vi "Set Zero Offset Mode.vi"(8 "error in (no error)":errorcluster, 9 "Reference Value (0.0)":dbl format="%.4f", 10 "Zero Offset Mode (F: Off)":bool, 11 "VISA resource name":refnum<visa-resource-name>) -> (0 "error out":errorcluster, 3 "VISA resource name out":refnum<visa-resource-name>)   [LabVIEW 2014, in "Fluke 5XXX Series Multicalibrators.lvlib"]
doc: "This VI zeros the pressure module or sets the zero offset for capacitance measurement using the oscilloscope option. For pressure measurments, if the pressure module is an absolute module, the reference parameter must be supplied.\n\nNote:\n\nThis VI is available only for instrument models 5500A and 5520A with oscilloscope option SC600 (SC1100) or option 700P (pressure modules)."
uses:
  Fluke 5XXX Series Multicalibrators.lvlib
panel:
  # "On"
  # "Off"
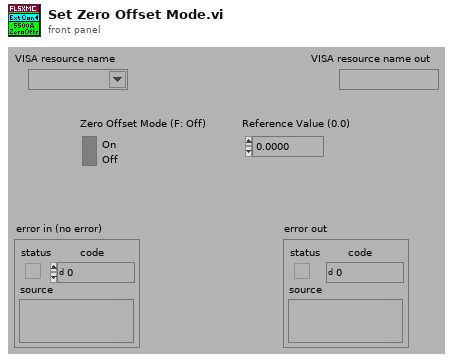
[diagram p1: front panel]
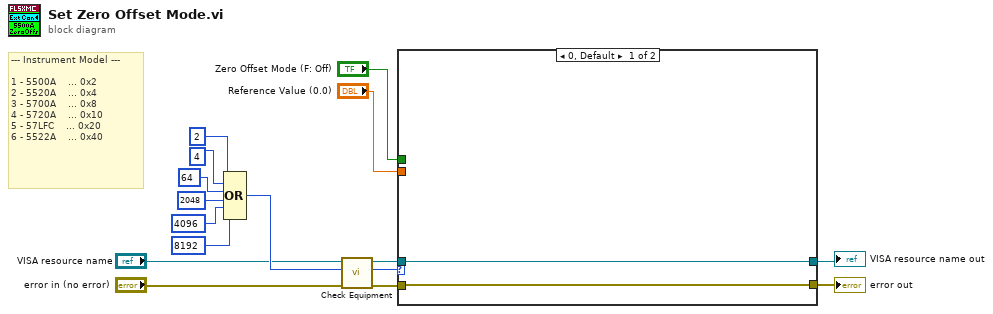
[diagram p0: block diagram]
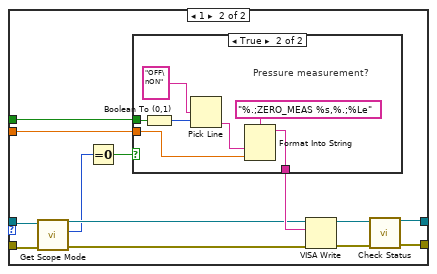
[diagram p2: hidden frame]
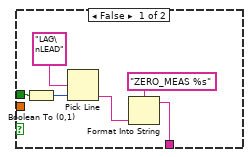
[diagram p3: hidden frame]
diagram:
  # "--- Instrument Model ---\n\n1 - 5500A    ... 0x2\n2 - 5520A    ... 0x4\n3 - 5700A    ... 0x8\n4 - 5720A    ... 0x10\n5 - 57LFC    ... 0x20\n6 - 5522A    ... 0x40"
  n1 = Compound Arithmetic op=OR(2 ("Numeric"), 4 ("Numeric"), 64 ("Numeric"), 2048 ("Numeric"), 4096 ("Numeric"), 8192 ("Numeric")) -> (w9:i32)
  n2 = call "Check Equipment.vi"("error in (no error)"="error in (no error)", "Bit Mask"=w9, "VISA resource name"="VISA resource name") -> ("error out"=w16:errorcluster, "Present?"=w15:u32, "VISA resource name out"=w14:refnum<visa-resource-name>)  [unwired: 6 in]
  n3 = case shown="0, Default" w15 {
    tunnel: [w17 w28] -> w4
    tunnel: w16 -> [w18 w23]
    tunnel: w14 -> [w17 w24]
    tunnel: [w18 w31] -> w5
    tunnel: "Zero Offset Mode (F: Off)" -> [_ w20]
    tunnel: "Reference Value (0.0)" -> [_ w19]
    frame 0, Default {
    }
    frame 1 {
      n4 = call "Get Scope Mode.vi"("error in (no error)"=w23, "VISA resource name"=w24) -> ("error out"=w26:errorcluster, "Scope Mode"=w22:i32, "VISA resource name out"=w25:refnum<visa-resource-name>)  [unwired: 7 in]
      n5 = Equal To 0?(x=w22) -> (x = 0?=w21:bool)
      n6 = case shown="True" w21 {
        tunnel: [w36 w38] -> w27
        tunnel: w20 -> [w33 w40]
        tunnel: w19 -> [_ w42]
        frame False {
          n7 = Boolean To (0,1)(Boolean=w33) -> (0, 1=w32:i16)
          n8 = Pick Line(multi-line string="LAG\nLEAD", line index=w32) -> (output string=w34:string)  [unwired: 1 in]
          n9 = Format Into String(format string="ZERO_MEAS %s", w34) -> (resulting string=w36:string)  [unwired: 2 in, 1 out]
        }
        frame True {
          # "Pressure measurement?"
          n10 = Boolean To (0,1)(Boolean=w40) -> (0, 1=w39:i16)
          n11 = Pick Line(multi-line string="OFF\nON", line index=w39) -> (output string=w41:string)  [unwired: 1 in]
          n12 = Format Into String(format string="%.;ZERO_MEAS %s,%.;%Le", w41, w42) -> (resulting string=w38:string)  [unwired: 2 in, 1 out]
        }
      }
      n13 = VISA Write(VISA resource name=w25, write buffer=w27, error in (no error)=w26) -> (VISA resource name out=w29:refnum<visa-resource-name>, error out=w30:errorcluster)  [unwired: 1 out]
      n14 = call "Check Status.vi"("VISA resource name"=w29, "error in (no error)"=w30) -> ("VISA resource name out"=w28:refnum<visa-resource-name>, "error out"=w31:errorcluster)  [unwired: 12 in]
    }
  }
  "VISA resource name out" <- w4
  "error out" <- w5
